vi "stopCI1_img.vi"   [LabVIEW 2013]
types:
  T1 = cluster{" CI1":refnum<k21>, "E_CI1":errorcluster}
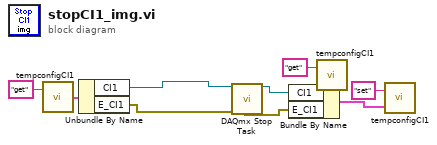
[diagram p0: block diagram]
diagram:
  n1 = call "tempconfigCI1.vi"("command"="get") -> ("Temp Config out"=w2:T1)  [unwired: 1 in]
  n2 = Unbundle By Name(w2) -> ("CI1"=w9:refnum<k21>, "E_CI1"=w10:errorcluster)
  n3 = call <vilib>:"DAQmx Stop Task.vi"("task/channels in"=w9, "error in"=w10) -> ("task out"=w7:refnum<k21>, "error out"=w8:errorcluster)  [unwired: 12 in]
  n4 = call "tempconfigCI1.vi"("command"="get") -> ("Temp Config out"=w5:T1)  [unwired: 1 in]
  n5 = Bundle By Name(cluster=w5, "CI1"=w7, "E_CI1"=w8) -> (w6:T1)
  n6 = call "tempconfigCI1.vi"("Temp Config in"=w6, "command"="set") -> ()  [unwired: 1 out]
